vi "initiateNotification.vi"(8 "error in (no error)":errorcluster, 11 "reference in":refnum<class "Project Panels.lvclass">) -> (0 "error out":errorcluster, 1 "table":cluster{"notification":string[][]}, 3 "reference out":refnum<class "Project Panels.lvclass">)   [LabVIEW 2014, in "Project Panels.lvclass"]
uses:
  Project Panels.lvclass
  SYS/Notification Controller_class/Notification Controller.lvclass
  APP/itemsNotification_class/itemsNotification.lvclass
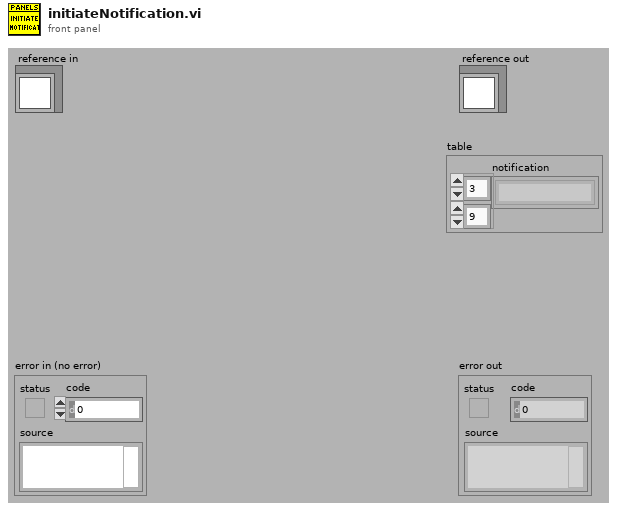
[diagram p1: front panel]
types:
  T1 = typedef "Project Panels.lvclass/ObjectAttributesRef.ctl" = refnum<data-value>
  T2 = typedef "Project Panels.lvclass/ObjectAttributes.ctl" = cluster{"MyAttribute":dbl, "device_controller_ref":refnum<class "Devices Controller.lvclass">, "file_controller_ref":refnum<class "File Controller.lvclass">, "item_controller_ref":refnum<class "Items Controller.lvclass">, "item_tables":cluster{"checkIN":string[][], "checkOUT":string[][], "storage":string[][]}, "quickbook_table":cluster{"notes":string[][]}, "notification_controller_ref":refnum<class "Notification Controller.lvclass">, "partstracking_controller_ref":refnum<class "PartsTracking Controller.lvclass">, "product_tables":cluster{"k4b2":string[][], "fitmate":string[][], "RMR":string[][], "CPET":string[][], "BP":string[][], "PP":string[][], "k5":string[][], "bb-pft":string[][]}, "rowsColour":u32[]}
  T3 = typedef "Devices Controller.lvclass/deviceType.ctl" = enum16{"k5", "k4b2", "fitmate", "cpet", "rmr", "bodyBoxPft", "bp", "pp"}
  T4 = cluster{"deviceType":T3, "S/N":string, "SW":string, "Description":string, "Account":string, "System's Location":string, "End User":string, "Email":string, "City":string, "LastChange":string, "Service By":string, "Exp Date":string, "FollowUp Sent":string, "FollowUp Accepted":string, "Note":string}
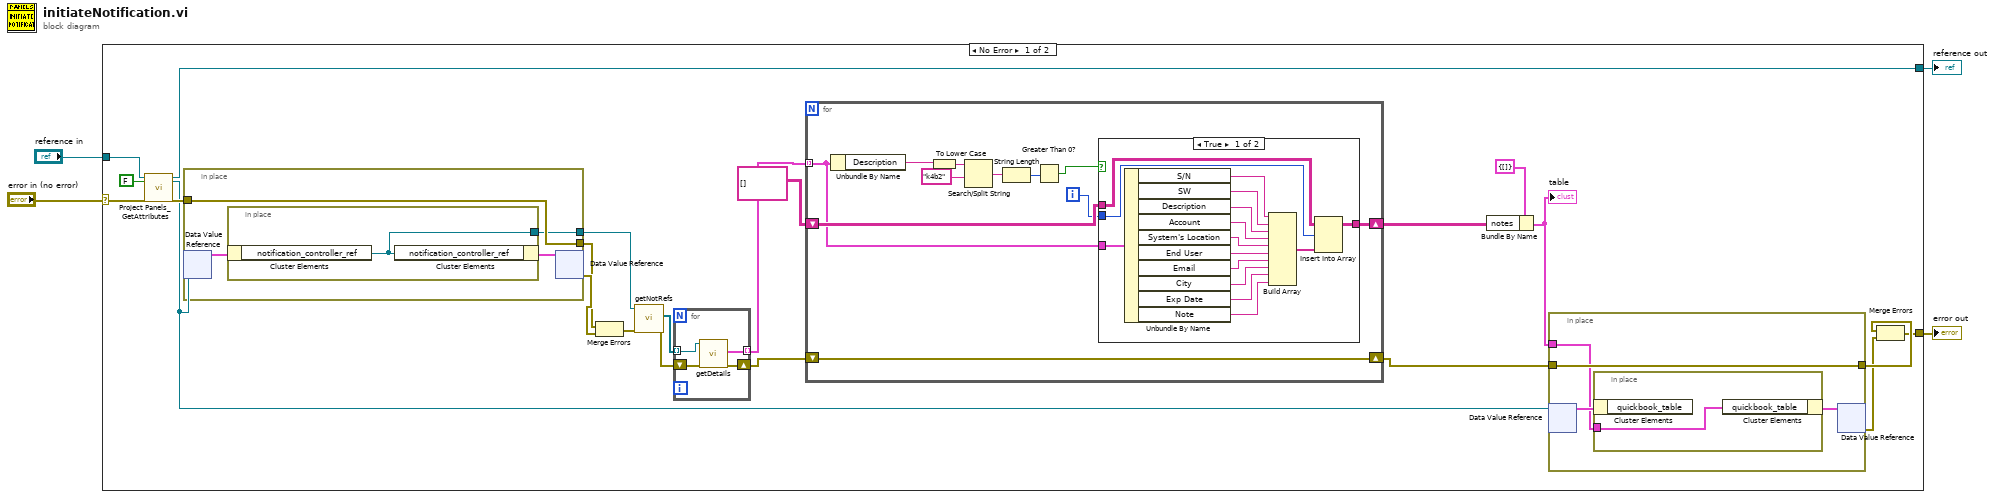
[diagram p0: block diagram]
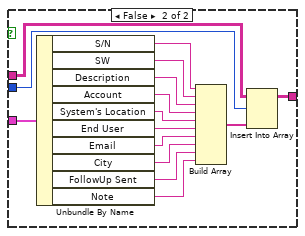
[diagram p2: hidden frame]
diagram:
  n1 = case shown="No Error" "error in (no error)" {
    selector: "error in (no error)" -> [w12 w83]
    tunnel: [w13 w83] -> w3
    tunnel: [w21 w82] -> w1
    tunnel: "reference in" -> [w24 w82]
    frame No Error {
      n2 = call "Project Panels_GetAttributes.vi"("reference in"=w24, "return data? (T)"=FALSE, "error in (no error)"=w12) -> ("reference out"=w21:refnum<class "Project Panels.lvclass">, "attributes ref"=w16:T1, "error out"=w22:errorcluster)  [unwired: 13 in, 1 out]
      n3 = in-place {
        in-place-border: w22 -> [w78]
        in-place-border: [w78] -> w25
        in-place-border: [w77] -> w11
        n4 = in-place-dvr #1(w16) -> (w79:T2)  [unwired: 1 out]
        n5 = in-place {
          in-place-border: [w81] -> w77
          n6 = in-place-cluster #2(w79) -> ("notification_controller_ref"=w81:refnum<class "Notification Controller.lvclass">)
          n7 = in-place-cluster #2("notification_controller_ref"=w81) -> (w80:T2)
        }
        n8 = in-place-dvr #1(w80) -> (w26:errorcluster)  [unwired: 1 out]
      }
      n9 = Merge Errors(w25, w26) -> (w20:errorcluster)
      n10 = call "getNotRefs.vi"("error in (no error)"=w20, "reference in"=w11) -> ("error out"=w17:errorcluster, "notification_refs"=w10:refnum<class "itemsNotification.lvclass">[])  [unwired: 6 in, 2 out]
      n11 = for {
        shift-right: [w34] -> w18
        shift-left: w17 -> [w35]
        tunnel: [w33] -> w19 mode=indexing
        tunnel: w10 -> [w32] mode=indexing
        n12 = call "getDetails.vi"("error in (no error)"=w35, "reference in"=w32) -> ("error out"=w34:errorcluster, "details"=w33:T4)  [unwired: 7 in, 1 out]
      }
      n13 = for {
        tunnel: w19 -> [w42] mode=indexing
        shift-right: [w45] -> w5
        shift-left: string[][] [] ("Table Control") -> [w46]
        shift-right: [w43] -> w7
        shift-left: w18 -> [w43]
        i -> [w44]
        n14 = Unbundle By Name(w42) -> ("Description"=w37:string)
        n15 = To Lower Case(string=w37) -> (all lower case string=w41:string)
        n16 = Search/Split String(string=w41, search string/char (-)="k4b2") -> (match + rest of string=w39:string)  [unwired: 1 in, 2 out]
        n17 = String Length(string=w39) -> (length=w38:i32)
        n18 = Greater Than 0?(x=w38) -> (x > 0?=w36:bool)
        n19 = case shown="True" w36 {
          tunnel: w46 -> [w61 w76]
          tunnel: [w60 w75] -> w45
          tunnel: w44 -> [w58 w73]
          tunnel: w42 -> [w47 w62]
          frame True {
            n20 = Unbundle By Name(w47) -> ("S/N"=w59:string, "SW"=w57:string, "Description"=w56:string, "Account"=w55:string, "System's Location"=w54:string, "End User"=w53:string, "Email"=w52:string, "City"=w51:string, "Exp Date"=w50:string, "Note"=w49:string)
            n21 = Build Array(w59, w57, w56, w55, w54, w53, w52, w51, w50, w49) -> (w48:string[])
            n22 = Insert Into Array(array=w61, index (row)=w58, new element=w48) -> (w60:string[][])  [unwired: 1 in]
          }
          frame False {
            n23 = Unbundle By Name(w62) -> ("S/N"=w74:string, "SW"=w72:string, "Description"=w71:string, "Account"=w70:string, "System's Location"=w69:string, "End User"=w68:string, "Email"=w67:string, "City"=w66:string, "FollowUp Sent"=w65:string, "Note"=w64:string)
            n24 = Build Array(w74, w72, w71, w70, w69, w68, w67, w66, w65, w64) -> (w63:string[])
            n25 = Insert Into Array(array=w76, index (row)=w73, new element=w63) -> (w75:string[][])  [unwired: 1 in]
          }
        }
      }
      n26 = Bundle By Name(cluster=cluster{"notes":string[][]} {"notes"=[]} ("quickbook_table"), "notes"=w5) -> (w6:cluster{"notes":string[][]})
      "table" <- w6
      n27 = in-place {
        in-place-border: w7 -> [w28]
        in-place-border: [w28] -> w15
        in-place-border: w6 -> [w27]
        n28 = in-place-dvr #3(w16) -> (w29:T2)  [unwired: 1 out]
        n29 = in-place {
          in-place-border: w27 -> [w31]
          n30 = in-place-cluster #4(w29) -> ()  [unwired: 1 out]
          n31 = in-place-cluster #4("quickbook_table"=w31) -> (w30:T2)
        }
        n32 = in-place-dvr #3(w30) -> (w14:errorcluster)  [unwired: 1 out]
      }
      n33 = Merge Errors(w15, w14) -> (w13:errorcluster)
    }
    frame Error {
    }
  }
  "error out" <- w3
  "reference out" <- w1
